vi "Convert Overrides.vi"(10 "Cluster":cluster{dbl[], bool[]}, 11 "Velocity (fps)":dbl) -> (3 "Array":T1(array[cluster]))   [LabVIEW 2019]
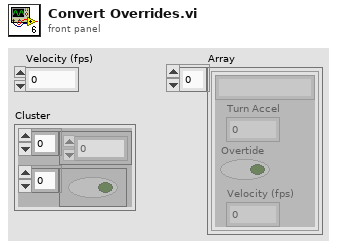
[diagram p1: front panel]
types:
  T1 = cluster{string, "Turn Accel":dbl, "Overtide":bool, "Velocity (fps)":dbl}[]
  T2 = cluster{string, "Angular Multiplier":dbl, "1":bool, "Velocity (fps)":dbl}
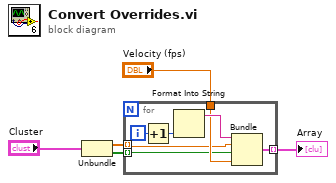
[diagram p0: block diagram]
diagram:
  n1 = Unbundle("Cluster") -> (w2:dbl[], w1:bool[])
  n2 = for {
    tunnel: [w12] -> w4 mode=indexing
    tunnel: "Velocity (fps)" -> [w9]
    tunnel: w2 -> [w8] mode=indexing
    tunnel: w1 -> [w7] mode=indexing
    i -> [w11]
    n3 = Increment(x=w11) -> (x+1=w6:i32)
    n4 = Format Into String(w6) -> (resulting string=w10:string)  [unwired: 3 in, 1 out]
    n5 = Bundle(w10, "Angular Multiplier"=w8, "1"=w7, "Velocity (fps)"=w9) -> (w12:T2)  [unwired: 1 in]
  }
  "Array" <- w4
